vi "Deactivate Subscription Policy.vi"(8 "error in (no error)":errorcluster, 11 "Subscription Policy":T1) -> (0 "error out":errorcluster)   [LabVIEW 2017, in "IMediator.lvlib" / "ISubscriptionPolicy.lvclass"]
doc: "This method decides whether or not to send or otherwise handle the new data value. The policy is set and maintained by the subscriber. The Topic Actor knows no policy details, it just passes the new value in. If there is a failure inside this method, the Topic Actor must assume the listener is no longer valid (dead/unrecoverable) and should delete it from the Subscriber list.\n\n<License>\nCopyright © 2017 Composed Systems, LLC | All rights reserved\nwww.composed.io\n\nAuthor: Ethan Stern <ethan.stern@composed.io>\n\nThis software is provided \"AS IS\" WITHOUT WARRANTIES, either express or implied, AND IS FOR EDUCATIONAL PURPOSES ONLY.\n</License>"
uses:
  ISubscriptionPolicy.lvclass
  ISubscriptionPolicy Reference.ctl
  ISubscriptionPolicy.lvclass/ISubscriptionPolicy.ctl
panel:
  out "Subscription Policy Out":T1
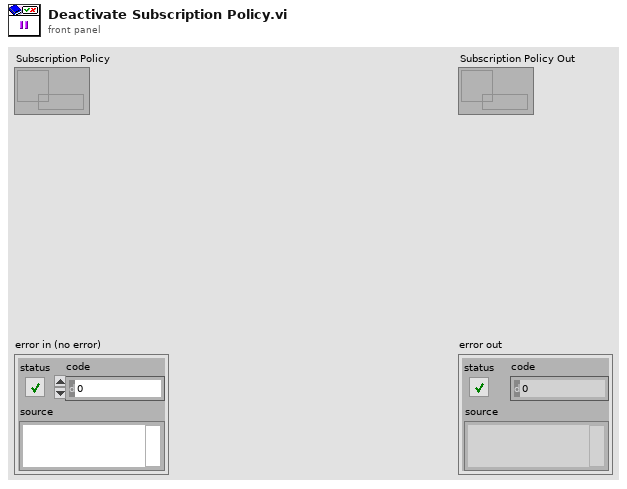
[diagram p1: front panel]
types:
  T1 = typedef "IMediator.lvlib/ISubscriptionPolicy.lvclass/ISubscriptionPolicy Reference.ctl" = refnum<data-value>
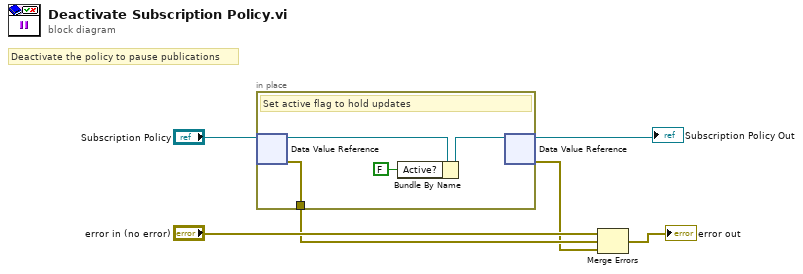
[diagram p0: block diagram]
diagram:
  # "Deactivate the policy to pause publications"
  n1 = in-place {
    in-place-border: [w9] -> w3
    # "Set active flag to hold updates"
    n2 = in-place-dvr #1("Subscription Policy") -> (w10:refnum<class "ISubscriptionPolicy.lvclass">, w9:errorcluster)
    n3 = Bundle By Name(cluster=w10, "Active?"=FALSE) -> (w8:refnum<class "ISubscriptionPolicy.lvclass">)
    n4 = in-place-dvr #1(w8) -> (→"Subscription Policy Out":T1, w2:errorcluster)
  }
  n5 = Merge Errors("error in (no error)", w3, w2) -> (→"error out":errorcluster)
